vi "Global_CMDShooter.vi"() -> ()   [LabVIEW 2017]
uses:
  Cluster_ShooterCMDInput.ctl
  Enum_ShooterCMDS.ctl
panel:
  in  "CMD Shooter":T1
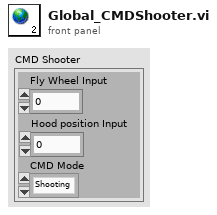
[diagram p1: front panel]
types:
  T1 = typedef "Cluster_ShooterCMDInput.ctl" = cluster{"Fly Wheel Input":dbl, "Hood position Input":dbl, "CMD Mode":T2}
  T2 = typedef "Enum_ShooterCMDS.ctl" = enum16{"Shooting", "Not Shooting"}
diagram:
